vi "Get_Temp_and_Press.vi"(4 "Averaging time (mins)":dbl=5.0 format="%.2f") -> (0 "Abs Press (mbar)":dbl format="%.2f", 2 "Temperature":dbl format="%.2f")   [LabVIEW 2020]
uses:
  ADAM Client/Sub VIs/Channel_State_Control.ctl
  Controls/Server_Comms.ctl
  ADAM Client/Sub VIs/ADAM Controls/Module_type_ADAM.ctl
  ADAM Client/Sub VIs/ADAM Controls/Calib_type_ADAM.ctl
  Controls/Global_mode.ctl
  ADAM Client/Sub VIs/ADAM Controls/Ch_description_ADAM.ctl
  ADAM Client/Sub VIs/ADAM Controls/Function_ADAM.ctl
  ADAM Client/Sub VIs/ADAM Controls/Channel_State.ctl
  ADAM Client/Sub VIs/ADAM Controls/Address.ctl
  ADAM Client/Sub VIs/ADAM Controls/Update_scan_value.ctl
  Globals/Preference_global.vi
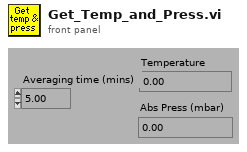
[diagram p1: front panel]
types:
  T1 = typedef "Channel_State_Control.ctl" = enum16{"Channel Name", "Channel Name Starts with", "Main Address"}
  T2 = typedef "Server_Comms.ctl" = enum16{"Server Link Healthy", "Do Not Link To Server"}
  T3 = typedef "Update_scan_value.ctl" = cluster{"Channel Name":string, "New Value":dbl}
  T4 = typedef "Ch_description_ADAM.ctl" = cluster{"Ch Name":string, "Type":T5, "Function":T6, "Ch State":T7, "Calibration type":T8, "A":dbl, "B":dbl, "C":dbl, "D":dbl, "Comments":string, "Address":T9, "String":string, "Duty":u16}
  T5 = typedef "Module_type_ADAM.ctl" = string
  T6 = typedef "Function_ADAM.ctl" = enum16{"Analogue Input", "Digital Input", "Event counter", "Event rate", "Analogue Output", "Digital Output", "Relay Output"}
  T7 = typedef "Channel_State.ctl" = enum16{"On", "Off", "Always On", "Always Off"}
  T8 = typedef "Calib_type_ADAM.ctl" = string
  T9 = typedef "Address.ctl" = cluster{"Main":i32, "Ch.":i32, "Sub":i32, "Port Name":string}
  T10 = typedef "Global_mode.ctl" = enum16{"Read Global", "Load Global From File", "Write Global to File"}
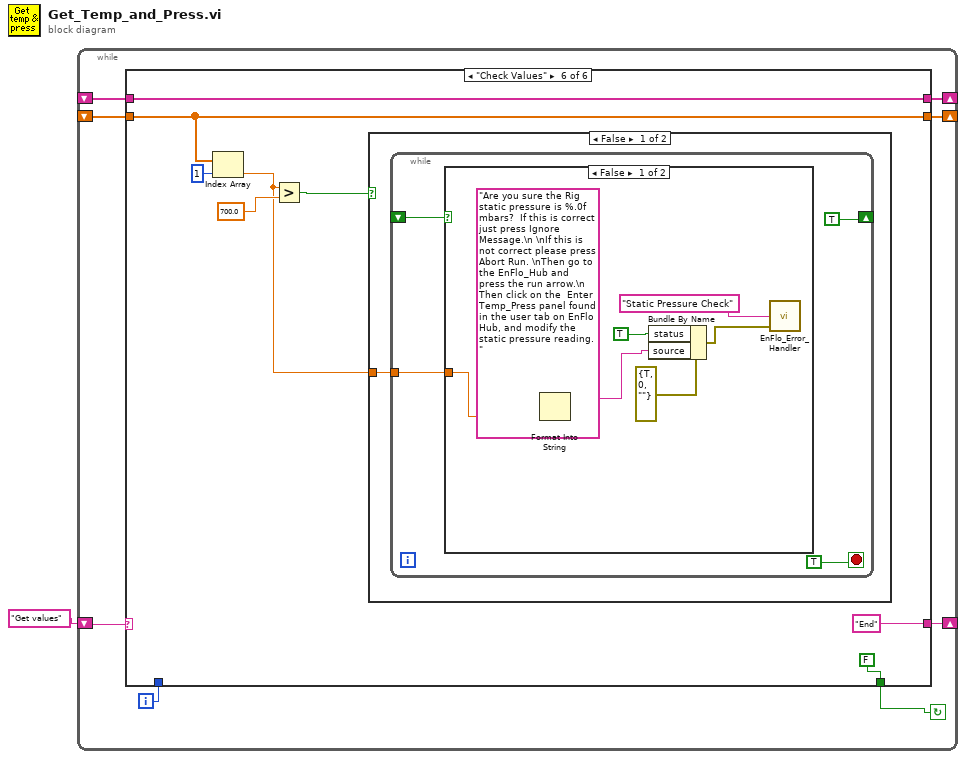
[diagram p0: block diagram]
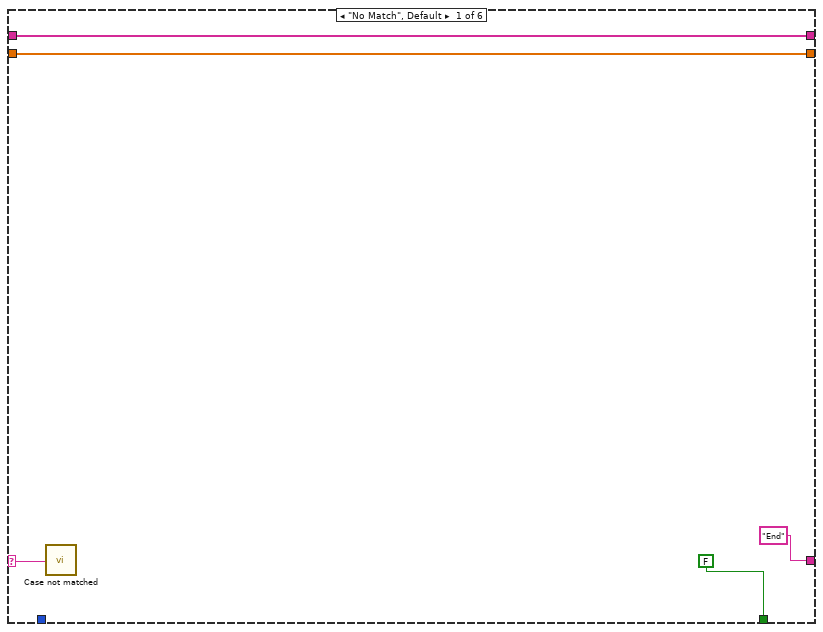
[diagram p2: hidden frame]
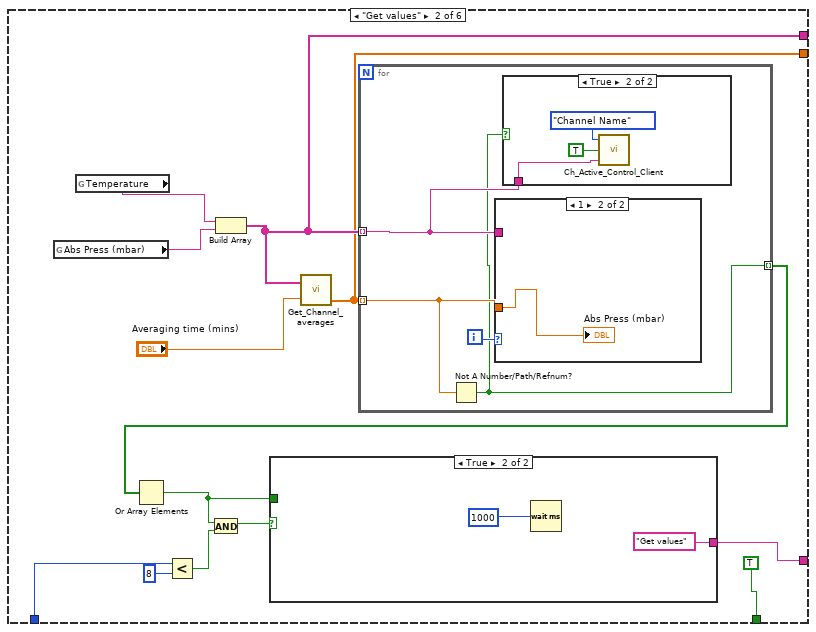
[diagram p3: hidden frame]
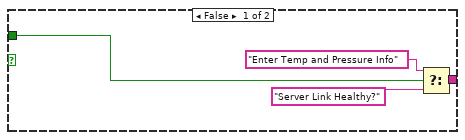
[diagram p4: hidden frame]
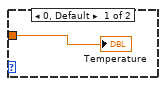
[diagram p6: hidden frame]
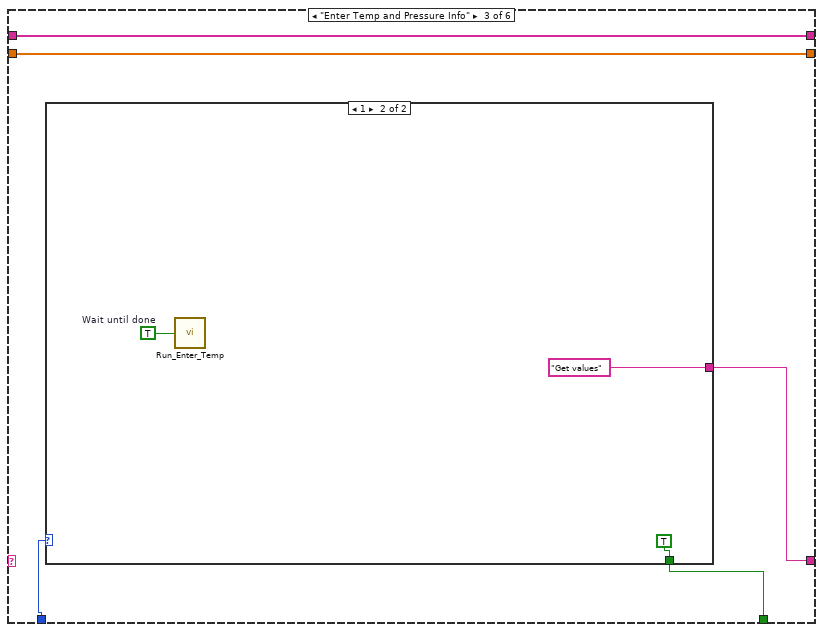
[diagram p7: hidden frame]
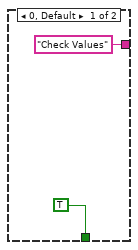
[diagram p8: hidden frame]
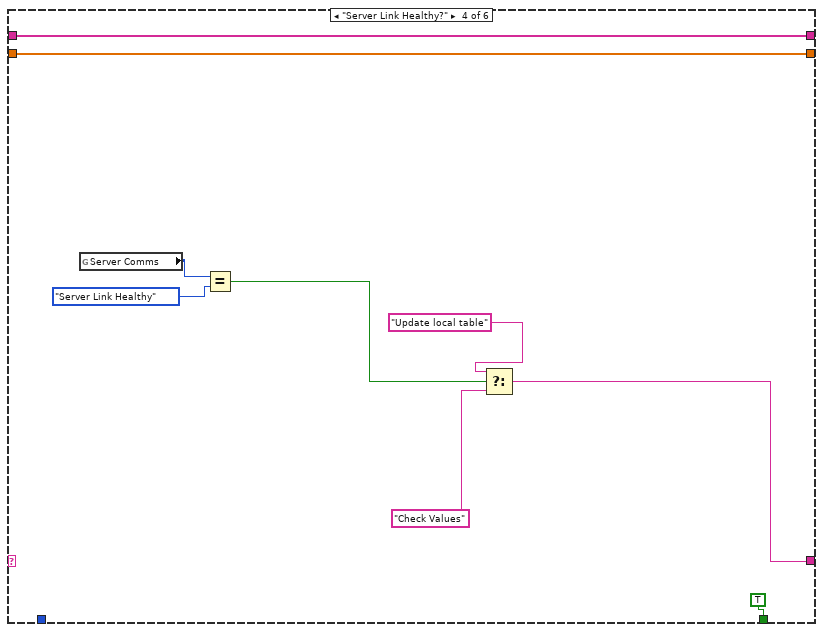
[diagram p9: hidden frame]
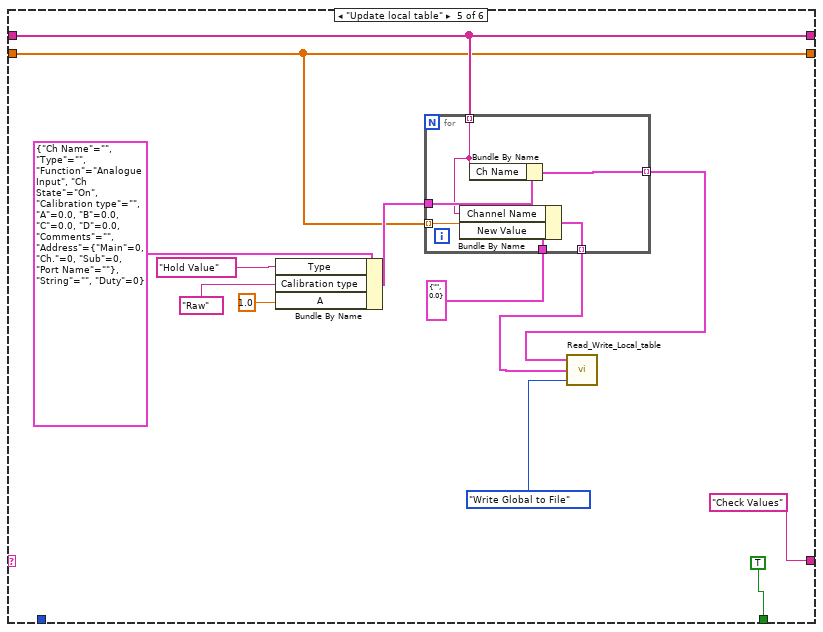
[diagram p10: hidden frame]
diagram:
  n1 = while {
    shift-right: [w8] -> _
    shift-left: "Get values" -> [w7]
    shift-right: [w6] -> _
    shift-left: _ -> [w4]
    shift-right: [w5] -> _
    shift-left: _ -> [w3]
    i -> [w2]
    stop <- w9 continue-if-true
    n2 = case shown="\"Check Values\"" w7 {
      selector: w7 -> [w10 _ _ _ _ _]
      tunnel: [FALSE TRUE w43 TRUE TRUE FALSE] -> w9
      tunnel: ["End" w22 w45 w55 "Check Values" "End"] -> w8
      tunnel: [w12 w21 w47 w61 w65 w86] -> w6
      tunnel: [w11 w20 w46 w60 w63 w85] -> w5
      tunnel: w4 -> [w12 _ w47 w61 w65 w86]
      tunnel: w3 -> [w11 _ w46 w60 w63 w85]
      tunnel: w2 -> [_ w19 w44 _ _ _]
      frame "No Match", Default {
        n3 = call "Case not matched.vi"("Case Name not Matched"=w10) -> ()
      }
      frame "Get values" {
        n4 = global read "Preference_global.vi" "Abs Press (mbar)"() -> (w27:string)
        n5 = global read "Preference_global.vi" "Temperature"() -> (w26:string)
        n6 = Less?(x=w19, y=8) -> (x < y?=w17:bool)
        n7 = Build Array(w26, w27) -> (w21:string[])
        n8 = call "Get_Channel_averages.vi"("Desired Ch Names"=w21, "Averaging time (mins)"="Averaging time (mins)") -> ("number"=w20:dbl[])  [unwired: 1 in, 2 out]
        n9 = for {
          tunnel: w21 -> [w35] mode=indexing
          tunnel: w20 -> [w36] mode=indexing
          tunnel: [w34] -> w23 mode=indexing
          i -> [w37]
          n10 = Not A Number/Path/Refnum?(number/path/refnum=w36) -> (NaN/Path/Refnum?=w34:bool)
          n11 = case shown="1" w37 {
            tunnel: w36 -> [w41 w42]
            tunnel: w35 -> [_ _]
            frame 0, Default {
              "Temperature" <- w41
            }
            frame 1 {
              "Abs Press (mbar)" <- w42
            }
          }
          n12 = case shown="True" w34 {
            tunnel: w35 -> [_ w38]
            frame False {
            }
            frame True {
              n13 = call "Ch_Active_Control_Client.vi"("Match"=w38, "Activate Channels?"=TRUE, "Control on"=Channel_State_Control."Channel Name") -> ()  [unwired: 2 out]
            }
          }
        }
        n14 = Or Array Elements(Boolean array=w23) -> (logical OR=w15:bool)
        n15 = And(x=w15, y=w17) -> (x .and. y?=w16:bool)
        n16 = case shown="True" w16 {
          tunnel: [w31 "Get values"] -> w22
          tunnel: w15 -> [w28 _]
          frame False {
            n17 = Select(t="Enter Temp and Pressure Info", s=w28, f="Server Link Healthy?") -> (s? t:f=w31:string)
          }
          frame True {
            n18 = Wait (ms)(milliseconds to wait=u32 1000 ("millisecond timer value")) -> ()  [unwired: 1 out]
          }
        }
      }
      frame "Enter Temp and Pressure Info" {
        n19 = case shown="1" w44 {
          tunnel: ["Check Values" "Get values"] -> w45
          tunnel: [TRUE TRUE] -> w43
          frame 0, Default {
          }
          frame 1 {
            w50 = TRUE  # Wait until done
            n20 = call "Run_Enter_Temp.vi"("Wait until done"=w50) -> ()  [unwired: 1 out]
          }
        }
      }
      frame "Server Link Healthy?" {
        n21 = global read "Preference_global.vi" "Server Comms"() -> (w58:T2)
        n22 = Equal?(x=w58, y=Server_Comms."Server Link Healthy" ("Server Comms")) -> (x = y?=w57:bool)
        n23 = Select(t="Update local table", s=w57, f="Check Values") -> (s? t:f=w55:string)
      }
      frame "Update local table" {
        n24 = Bundle By Name(cluster=T4 {"Ch Name"="", "Type"="", "Function"=enum."Analogue Input", "Ch State"=enum."On", "Calibration type"="", "A"=0.0, "B"=0.0, "C"=0.0, "D"=0.0, "Comments"="", "Address"={"Main"=0, "Ch."=0, "Sub"=0, "Port Name"=""}, "String"="", "Duty"=0} ("Ch Discription"), "Type"=T5 "Hold Value", "Calibration type"=T8 "Raw", "A"=1.0) -> (w68:T4)
        n25 = for {
          tunnel: w68 -> [w80]
          tunnel: [w79] -> w66 mode=indexing
          tunnel: w65 -> [w77] mode=indexing
          tunnel: T3 {"Channel Name"="", "New Value"=0.0} ("Update Scan Value Cluster") -> [w78]
          tunnel: w63 -> [w76] mode=indexing
          tunnel: [w75] -> w62 mode=indexing
          n26 = Bundle By Name(cluster=w78, "Channel Name"=w77, "New Value"=w76) -> (w75:T3)
          n27 = Bundle By Name(cluster=w80, "Ch Name"=w77) -> (w79:T4)
        }
        n28 = call "Read_Write_Local_table.vi"("Mode"=Global_mode."Write Global to File", "Ch Values in"=w62, "Channels Descriptions In"=w66) -> ()  [unwired: 3 out]
      }
      frame "Check Values" {
        n29 = Index Array(array=w85, index=1) -> (element=w81:dbl)
        n30 = Greater?(x=w81, y=700.0) -> (0:w82:bool)
        n31 = case shown="False" w82 {
          tunnel: w81 -> [w89 _]
          frame False {
            n32 = while {
              shift-right: [TRUE] -> _
              shift-left: _ -> [w92]
              tunnel: w89 -> [w91]
              stop <- TRUE stop-if-true
              n33 = case shown="False" w92 {
                tunnel: w91 -> [w96 _]
                frame False {
                  n34 = Format Into String(format string="Are you sure the Rig static pressure is %.0f mbars?  If this is correct just press Ignore Message.\n \nIf this is not correct please press Abort Run. \nThen go to the EnFlo_Hub and press the run arrow.\n Then click on the  Enter Temp_Press panel found in the user tab on EnFlo Hub, and modify the static pressure reading.", w96) -> (resulting string=w94:string)  [unwired: 2 in, 1 out]
                  n35 = Bundle By Name(cluster=errorcluster {"status"=TRUE, "code"=0, "source"=""} ("error in (no error)"), "status"=TRUE, "source"=w94) -> (w99:errorcluster)
                  n36 = call "EnFlo_Error_Handler.vi"("error in (no error)"=w99, "Error Type"="Static Pressure Check") -> ()  [unwired: 1 in, 3 out]
                }
                frame True {
                }
              }
            }
          }
          frame True {
          }
        }
      }
    }
  }
